vi "Write Controller Name.vi"(10 "控制器名称":string, 11 "定时循环控制器输入":refnum<class "Timed Loop Actor.lvclass">) -> (3 "定时循环控制器输出":refnum<class "Timed Loop Actor.lvclass">)   [LabVIEW 2015, in "Timed Loop Actor.lvlib" / "Timed Loop Actor.lvclass"]
doc: "写入控制器名称。实时系统中名称作为框架的一部分用于使定时循环停止执行，其他情况下名称仅用于调试。"
uses:
  Timed Loop Actor.lvclass
  Timed Loop Actor.lvclass/Timed Loop Actor.ctl
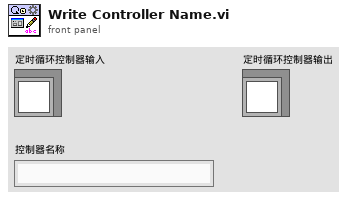
[diagram p1: front panel]
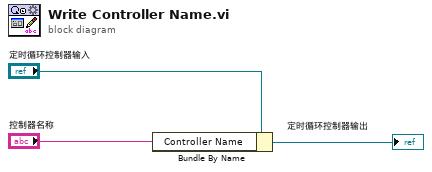
[diagram p0: block diagram]
diagram:
  n1 = Bundle By Name(cluster="定时循环控制器输入", "Controller Name"="控制器名称") -> (→"定时循环控制器输出":refnum<class "Timed Loop Actor.lvclass">)
